vi "TextFit_Get Characters Priority and Index.vi"(8 "Error":errorcluster, 11 "Char":T1) -> (0 "Error Out":errorcluster, 2 "Index Out":i32, 3 "Priority Out":i32)   [LabVIEW 2014]
doc: "Finds the Priority and Index of the input character"
uses:
  Controls/String_Picture/String Char Normal.ctl
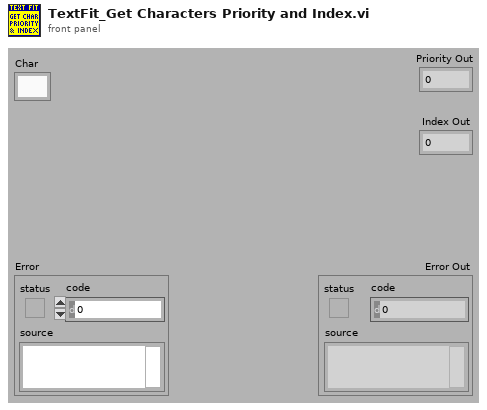
[diagram p1: front panel]
types:
  T1 = typedef "String Char Normal.ctl" = string
  T2 = typedef "Cluster_Font Data.ctl" = cluster{"Font List Out":T3[], "Char Array":T1[], "Seperator Index":i32}
  T3 = typedef "Cluster_Character Data.ctl" = cluster{"Char":T1, "Wide":T4, "Med":T5, "Thin":T6, "Priority":i32}
  T4 = typedef "Array Bool Char Bits Wide.ctl" = bool[][]
  T5 = typedef "Array Bool Char Bits Med.ctl" = bool[][]
  T6 = typedef "Array Bool Char Bits Thin.ctl" = bool[][]
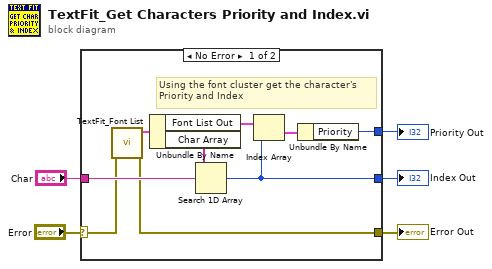
[diagram p0: block diagram]
diagram:
  n1 = case shown="No Error" "Error" {
    selector: "Error" -> [w6 w15]
    tunnel: [w14 _] -> w5
    tunnel: [w12 _] -> w4
    tunnel: "Char" -> [w9 _]
    tunnel: [w7 w15] -> w2
    frame No Error {
      # "Using the font cluster get the character's \nPriority and Index"
      n2 = call "TextFit_Font List.vi"("Error In"=w6) -> ("Error Out"=w7:errorcluster, "Font Cluster Out"=w8:T2)  [unwired: 9 in]
      n3 = Unbundle By Name(w8) -> ("Font List Out"=w11:T3[], "Char Array"=w10:T1[])
      n4 = Search 1D Array(1D array=w10, element=w9) -> (index of element=w12:i32)  [unwired: 1 in]
      n5 = Index Array(array=w11, index=w12) -> (element=w13:T3)
      n6 = Unbundle By Name(w13) -> ("Priority"=w14:i32)
    }
    frame Error {
    }
  }
  "Priority Out" <- w5
  "Index Out" <- w4
  "Error Out" <- w2
